vi "Plot PieChart.vi"(10 "Label":string[](array[string])) -> (1 "Labelling":cluster{dbl, "String":string}[](array[cluster]))   [LabVIEW 2017]
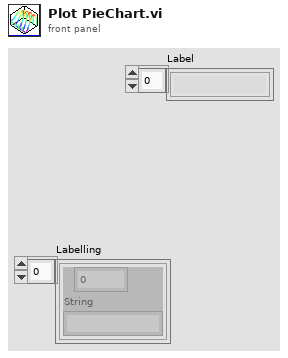
[diagram p1: front panel]
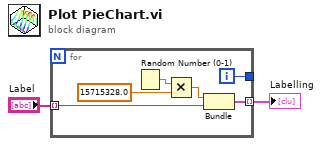
[diagram p0: block diagram]
diagram:
  n1 = for {
    tunnel: "Label" -> [w6] mode=indexing
    tunnel: [w5] -> w1 mode=indexing
    tunnel: [w3] -> _
    i -> [w3]
    n2 = Random Number (0-1)() -> (number: 0 to 1=w8:dbl)
    n3 = Multiply(x=w8, y=15715328.0) -> (x*y=w4:dbl)
    n4 = Bundle(w4, "String"=w6) -> (w5:cluster{dbl, "String":string})  [unwired: 1 in]
  }
  "Labelling" <- w1
